vi "GUI_HTT_Switcher.vi"() -> ()   [LabVIEW 2013]
uses:
  Shared/GUI_Template/GUI_master/tcp_new_data_event.ctl
  Shared/GUI_Template/GUI_master/tcp new data cluster.ctl
panel:
  in  "DigitalOutput.Channel 2::1":enum16{"on", "off"}(ring) caption="Phosphor"
  in  "Phosphor":bool
  in  "DigitalOutput.Channel 1::1":enum16{"on", "off"}(ring)
  in  "DigitalOutput.Channel 0::1":enum16{"on", "off"}(ring) caption="Flipper"
  in  "Flipper":bool
  out "error IO 2":errorcluster
  out "fire::10":string
  out "tcp data event":T1
  in  "UDP error message":string
  in  "GUIdevice 2":string
  in  "GUIdevice 1":string="HTT-Switch-DAQPad"
  in  "stop":bool
  # "Energy"
  # "HTT Switcher"
  # "In"
  # "Out"
  # "In"
  # "Out"
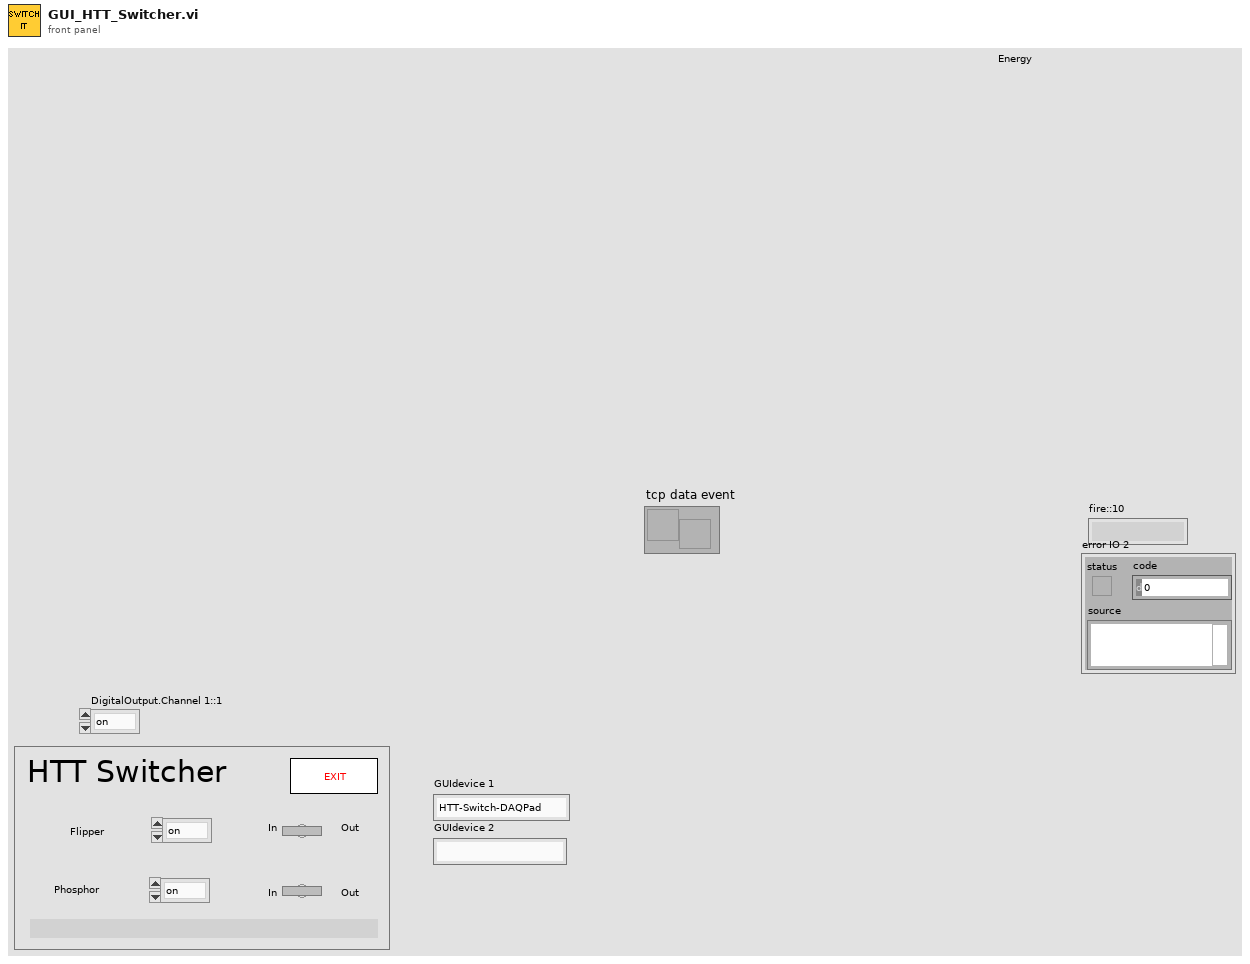
[diagram p1: front panel]
types:
  T1 = typedef "tcp_new_data_event.ctl" = refnum<user-event>
  T2 = typedef "tcp new data cluster.ctl" = cluster{"EventEnum":enum16{"new data", "connection status update"}, "Device name":string}
  T3 = enum32{"invalid app kind", "Development System", "Run Time System", "Student Edition", "Embedded LabVIEW", "Evaluation", "Custom"}
  T4 = enum32{"Invalid", "Standard", "Closed", "Hidden", "Minimized", "Maximized"}
  T5 = cluster{"Core":cluster{"Current VI Reference":refnum<vi>, "Close Panel on Exit?":bool}, "Heater timing offset":dbl, "Discharge timing offset":dbl, "Flipper":bool, "Tik1":u32, "Tik2":u32, "Flipperi":bool, "Phosphor":bool, "DigitalOutput.Channel 2::1":enum16{"on", "off"}}
  T6 = cluster{"Current VI Reference":refnum<vi>, "Close Panel on Exit?":bool}
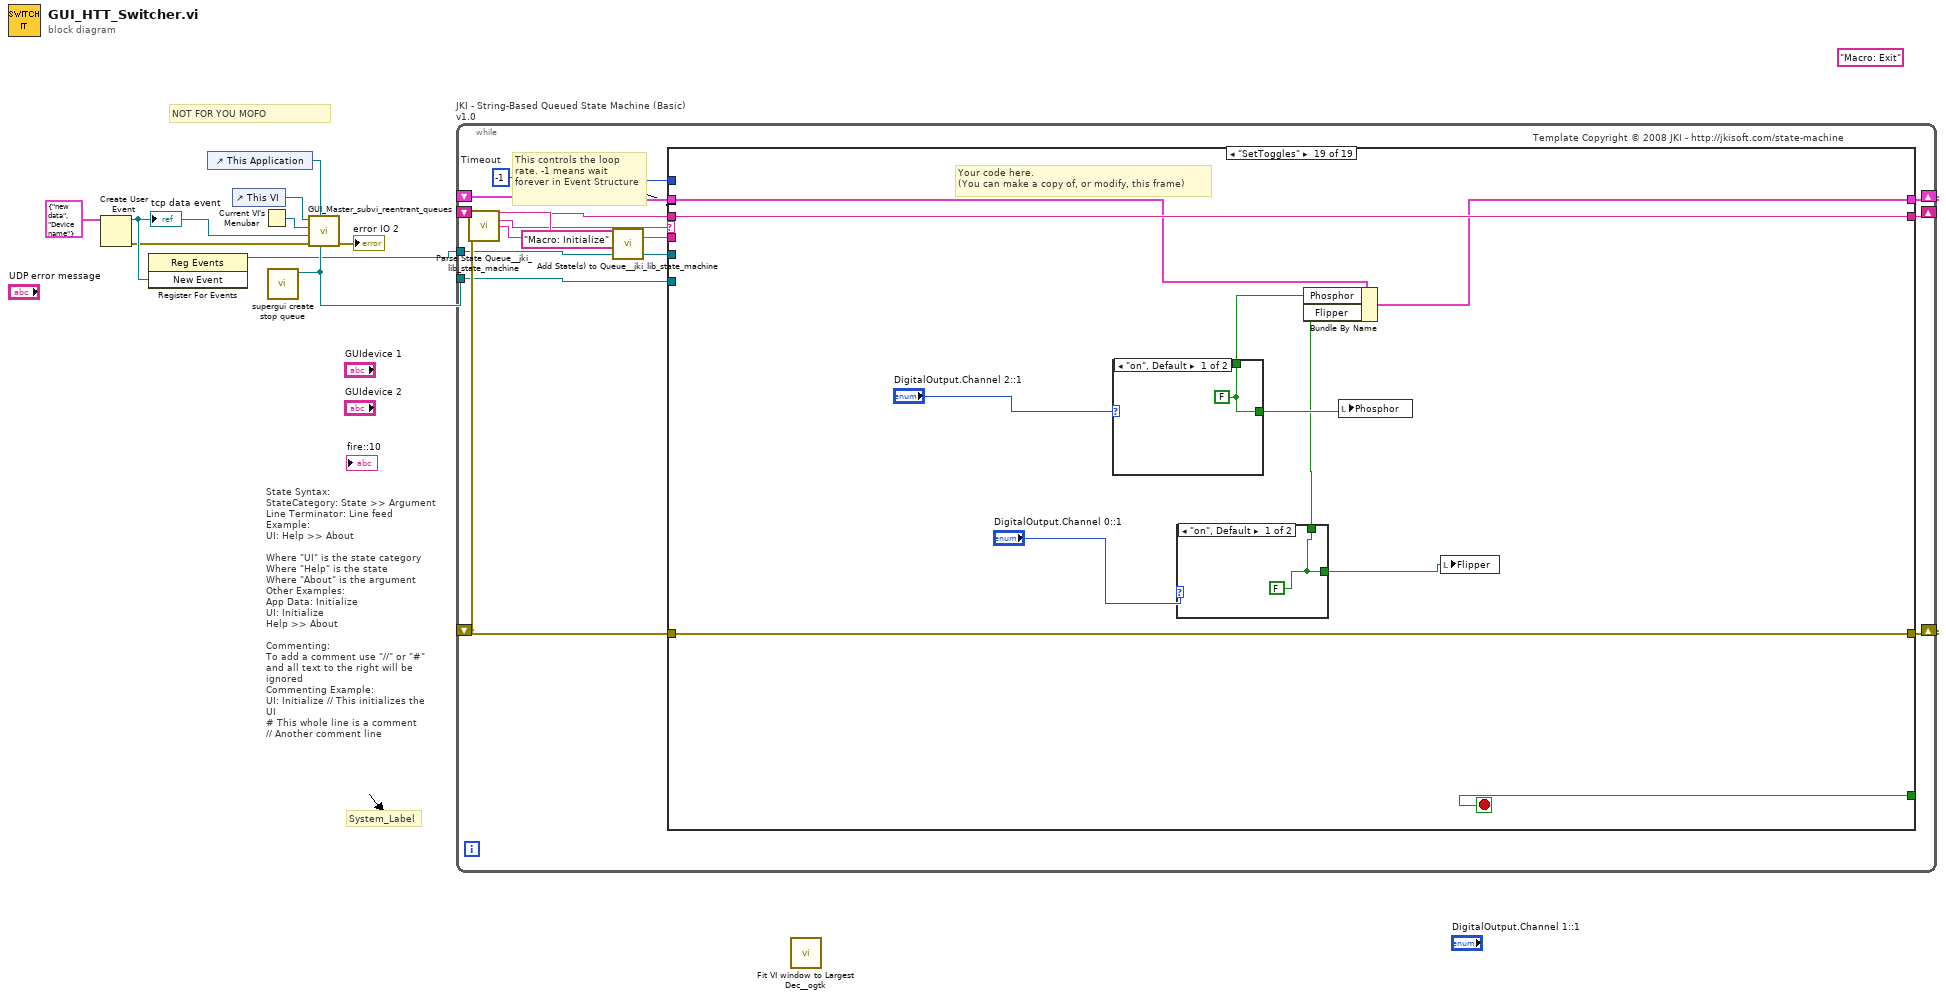
[diagram p0: block diagram]
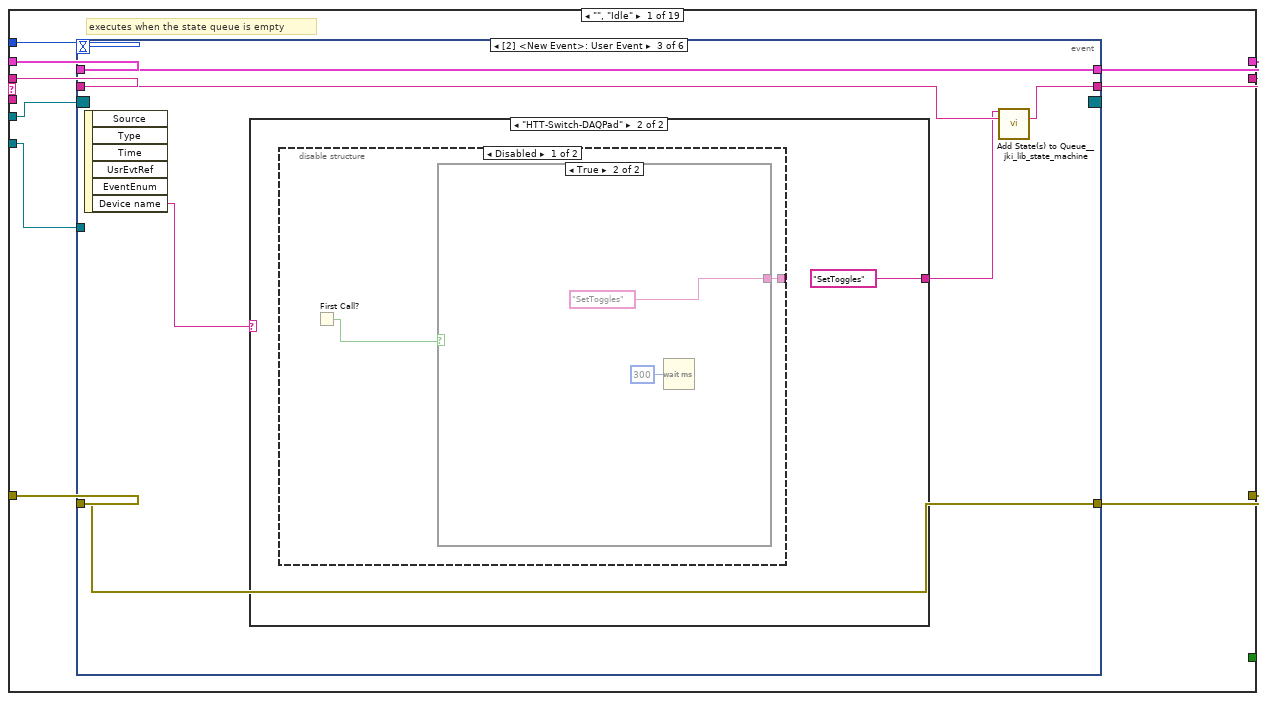
[diagram p2: hidden frame]
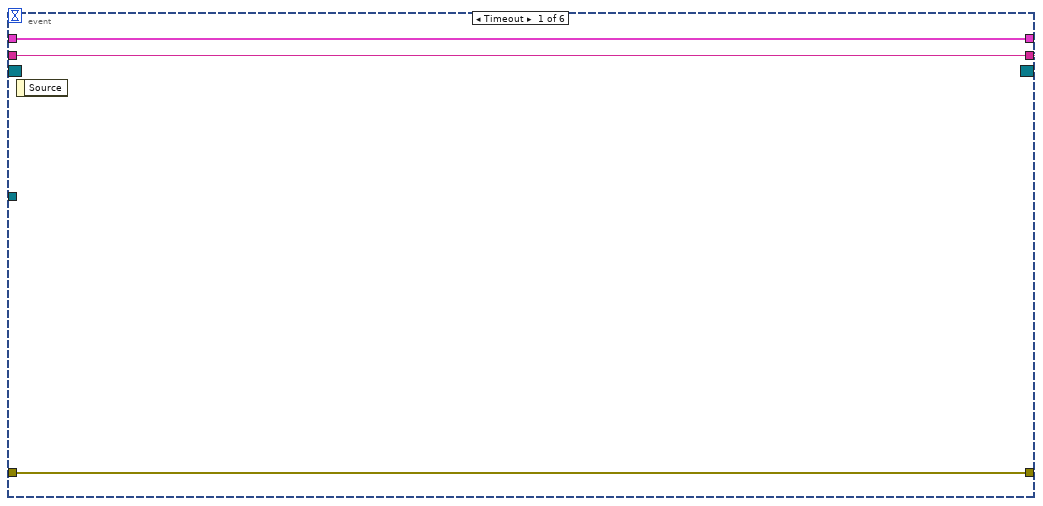
[diagram p3: hidden frame]
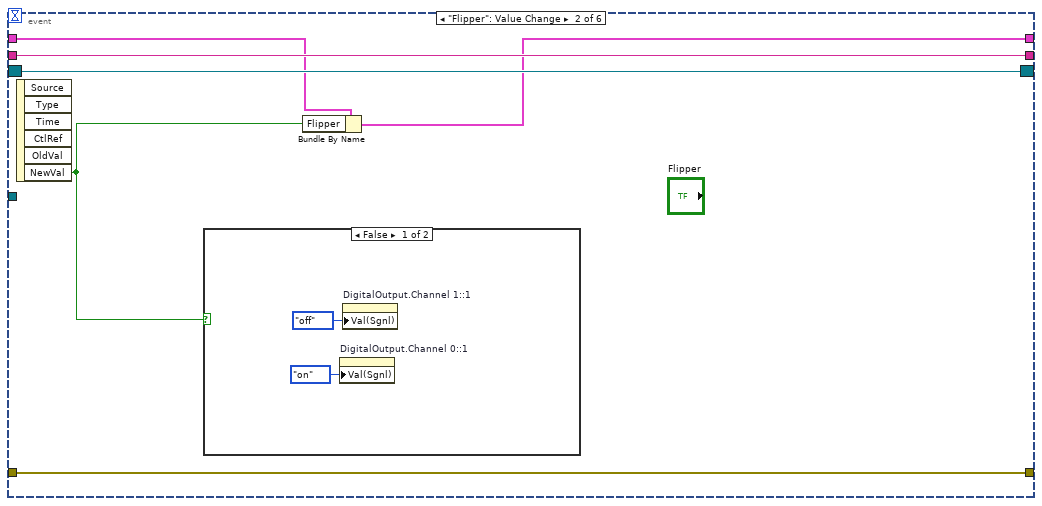
[diagram p4: hidden frame]
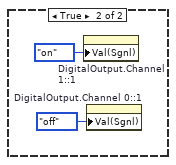
[diagram p5: hidden frame]
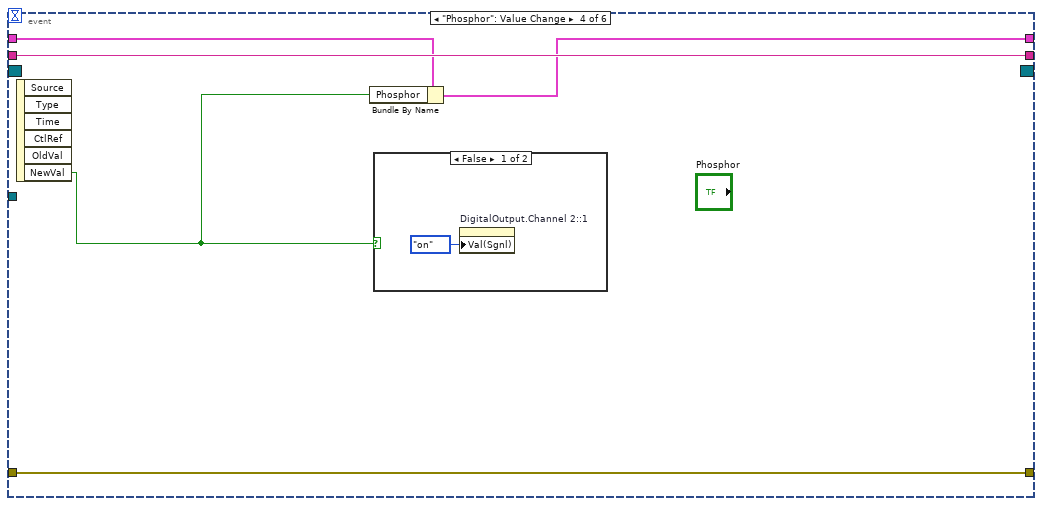
[diagram p9: hidden frame]
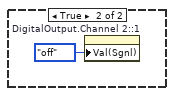
[diagram p10: hidden frame]
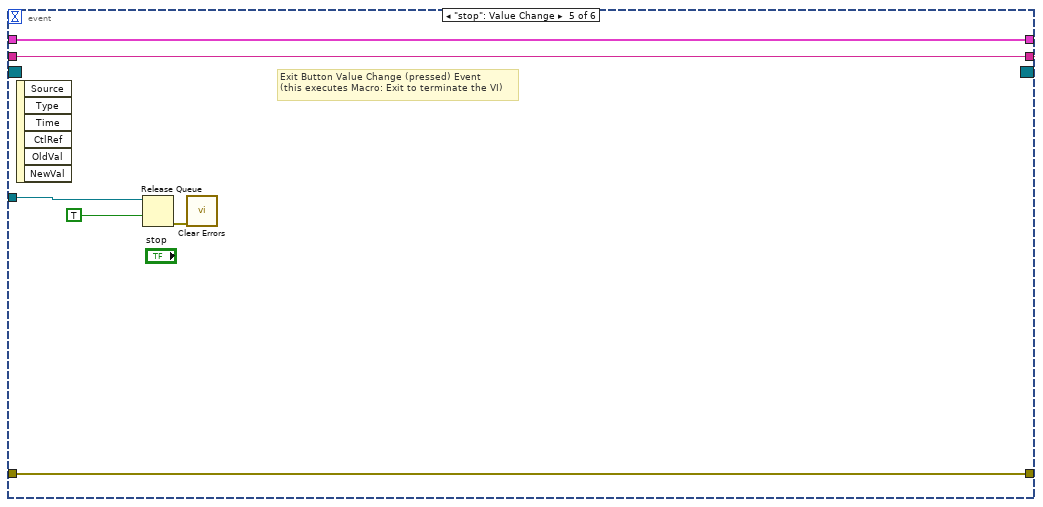
[diagram p11: hidden frame]
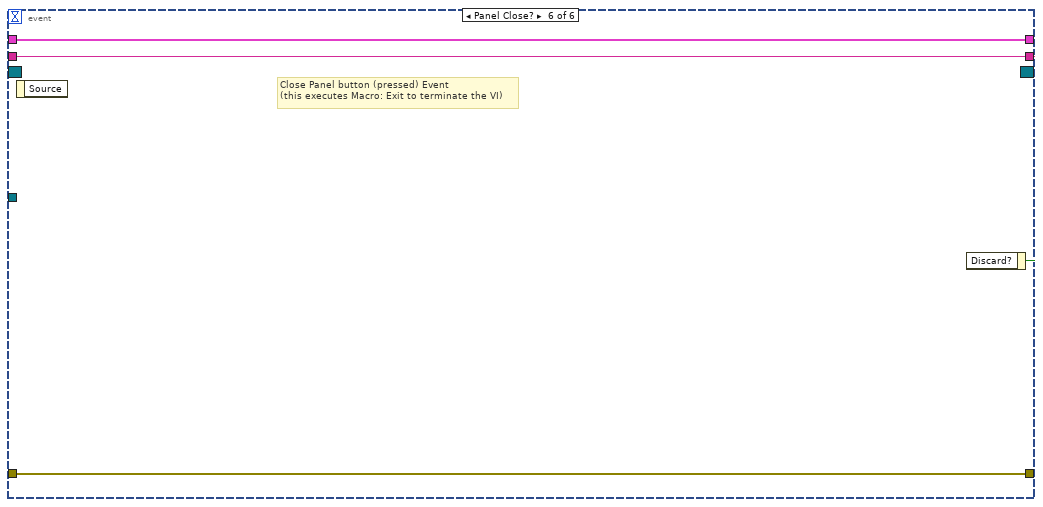
[diagram p12: hidden frame]
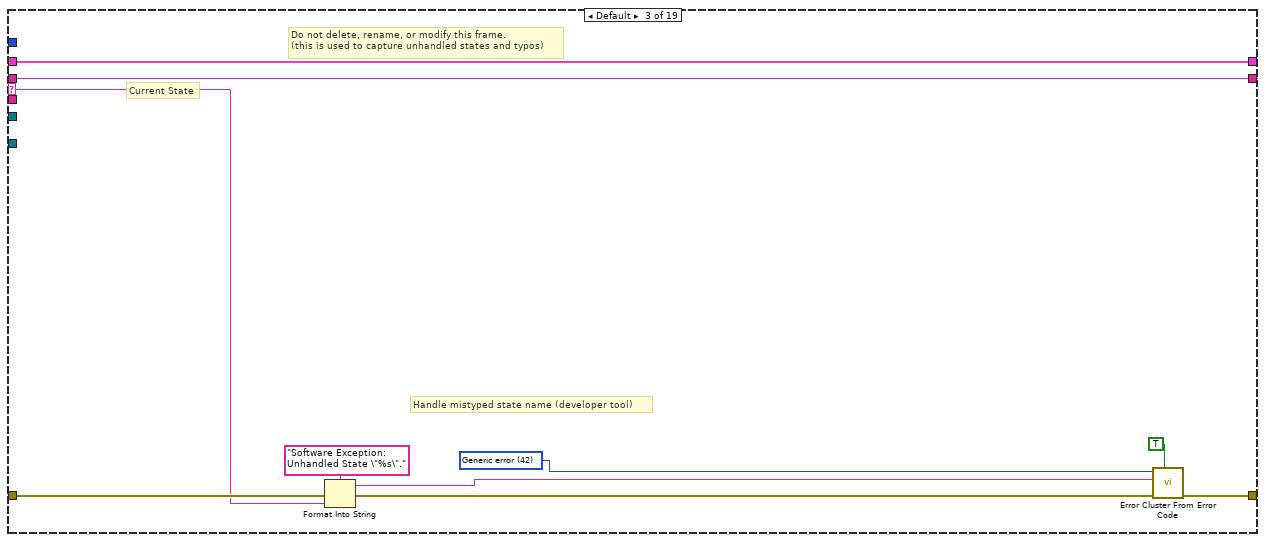
[diagram p14: hidden frame]
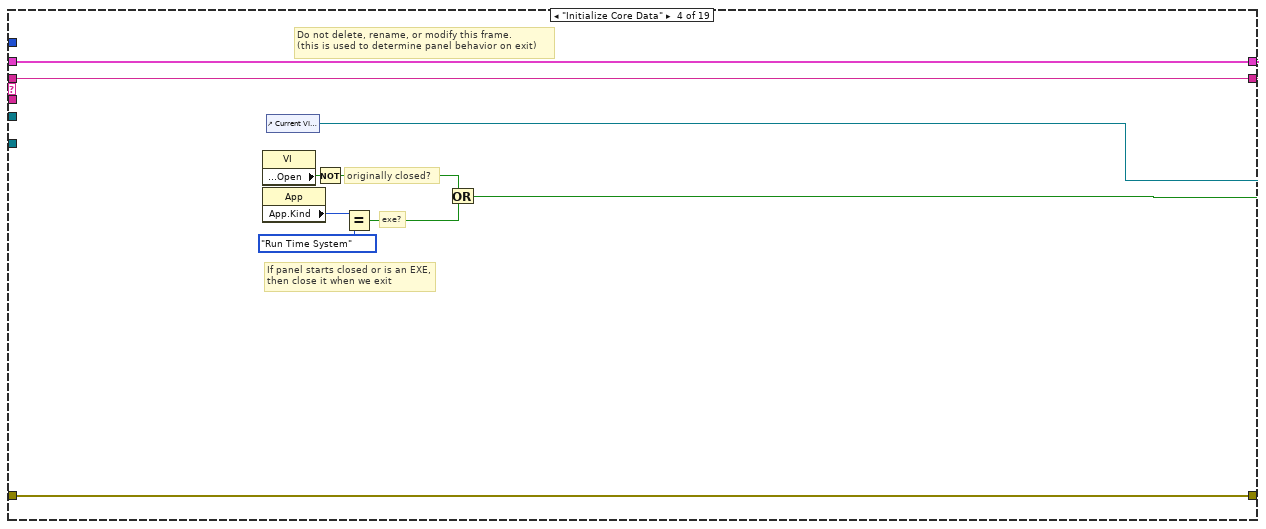
[diagram p15: hidden frame]
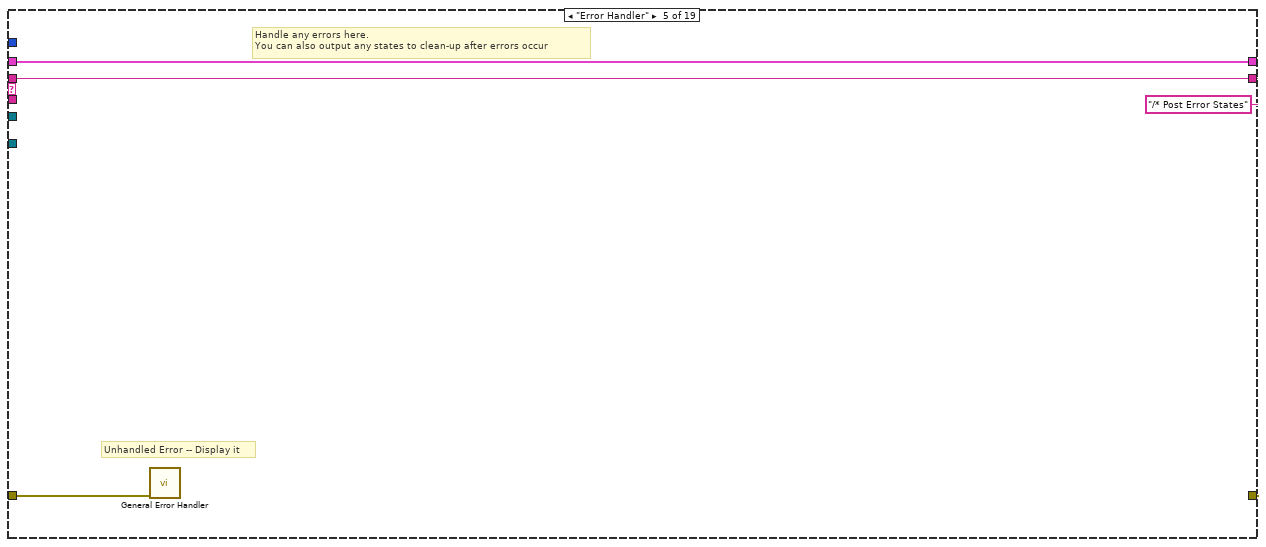
[diagram p16: hidden frame]
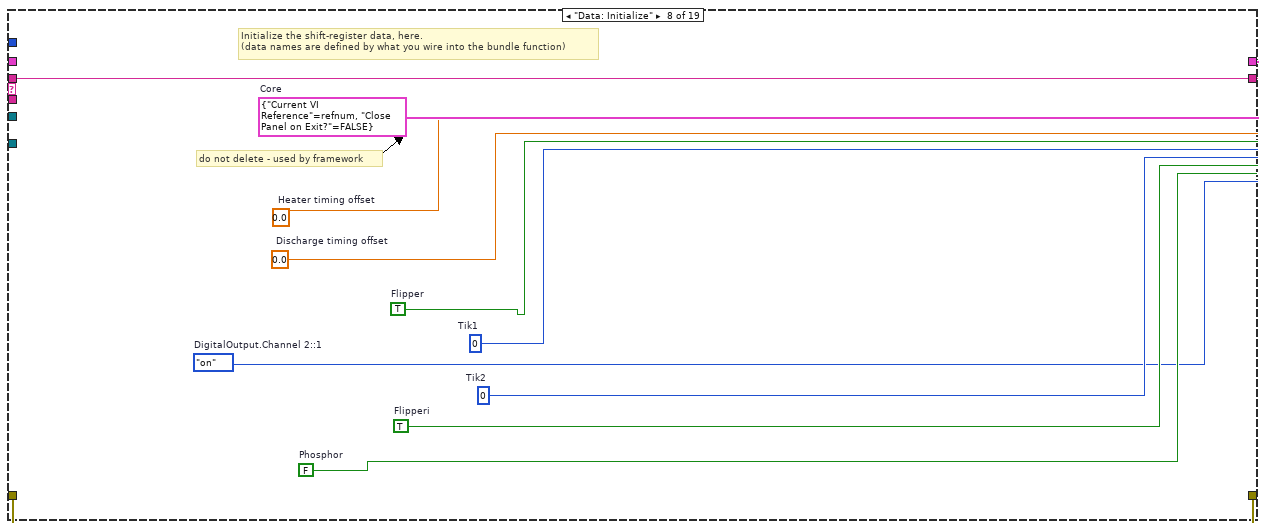
[diagram p19: hidden frame]
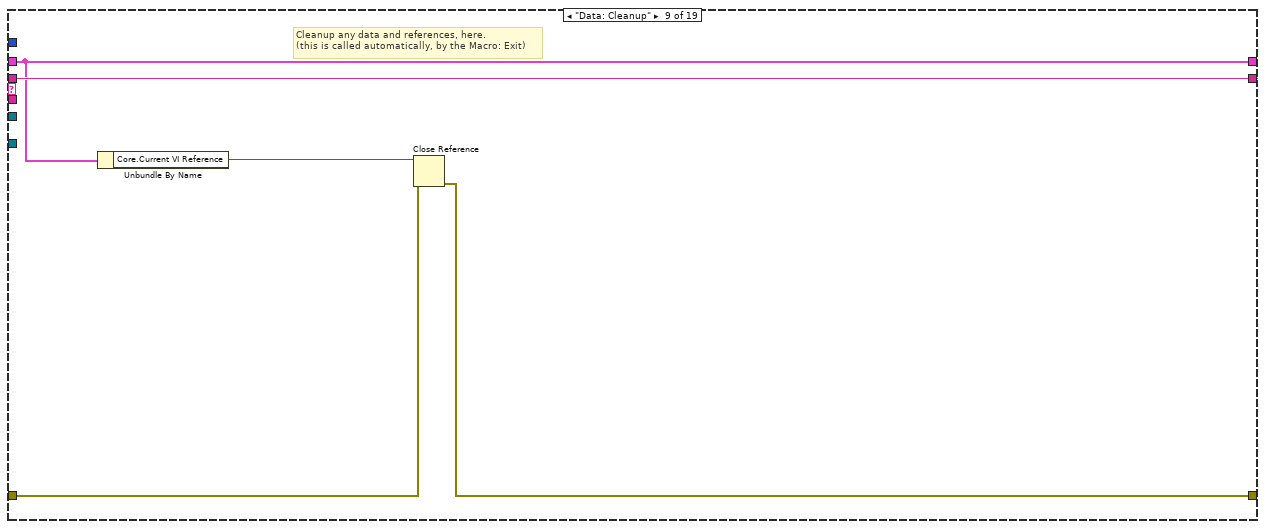
[diagram p20: hidden frame]
diagram:
  (unwired) "Macro: Exit"
  # "State Syntax:\nStateCategory: State >> Argument\nLine Terminator: Line feed\nExample:\nUI: Help >> About\n\nWhere \"UI\" is the state category\nWhere \"Help\" is the state\nWhere \"About\" is the argument\nOther Examples:\nApp Data: Initialize\nUI: Initialize\nHelp >> About\n\nCommenting:\nTo add a comment use \"//\" or \"#\" and all text to the right will be ignored\nCommenting Example:\nUI: Initialize // This initializes the UI\n# This whole line is a comment\n// Another comment line"
  # "This controls the loop rate. -1 means wait forever in Event Structure"
  # "System_Label"
  # "NOT FOR YOU MOFO"
  n1 = Create User Event(user event datatype=T2 {"EventEnum"=enum."new data", "Device name"="Device name"} ("New Event")) -> (user event=w10:refnum<user-event>, error out=w9:errorcluster)  [unwired: 1 in]
  "tcp data event" <- w10
  n2 = register-events(w10) -> (reference out=w1:refnum<event-registration>)  [unwired: 2 in, 1 out]
  n3 = control-ref of="This Application"() -> (w11:refnum<vi>)
  n4 = control-ref of="This VI"() -> (w5:refnum<vi>)
  n5 = Current VI's Menubar() -> (w7:refnum<k9>)
  n6 = call "supergui create stop queue.vi"() -> ("STOP Queue out"=w2:refnum<queue>)  [unwired: 11 in]
  n7 = call "GUI_Master_subvi_reentrant_queues.vi"("STOP Queue in"=w2, "This Application"=w11, "error in (no error)"=w9, "tcp data event"=w10, "Caller menu reference"=w7, "Caller VI ref"=w5) -> ("error out"=→"error IO 2":errorcluster)  [unwired: 5 in]
  n8 = call <vilib>:"Add State(s) to Queue__jki_lib_state_machine.vi"("State(s) in (\"\")"="Macro: Initialize") -> ("States Out"=w3:string)  [unwired: 14 in]
  n9 = while "JKI - String-Based Queued State Machine (Basic) v1.0" {
    shift-right: [w17] -> _
    shift-left: _ -> [w16]
    shift-right: [w20] -> _
    shift-left: _ -> [w14]
    shift-right: [w19] -> _
    shift-left: w3 -> [w21]
    tunnel: w1 -> [w13]
    tunnel: w2 -> [w12]
    stop <- w18 stop-if-true
    w15 = -1  # Timeout
    # "Template Copyright © 2008 JKI - http://jkisoft.com/state-machine"
    n10 = call <vilib>:"Parse State Queue__jki_lib_state_machine.vi"("State Queue"=w21, "Error In (no error)"=w14) -> ("Remaining States"=w23:string, "Current State"=w24:string, "Arguments"=w22:string)  [unwired: 11 in]
    n11 = case shown="\"SetToggles\"" w24 {
      selector: w24 -> [_ _ w84 _ _ _ _ _ _ _ _ _ _ _ _ _ _ _ _]
      tunnel: w23 -> [w33 w83 w88 w106 w112 w117 w121 w134 w140 w144 w148 w154 w165 w191 w196 w206 w210 w216 w227]
      tunnel: w22 -> [_ _ _ _ _ _ _ _ _ _ _ w149 w159 _ _ _ _ _ _]
      tunnel: w16 -> [w31 w80 w86 w97 w109 w115 w118 _ w135 w141 w146 w152 w161 w188 w192 w203 w207 w214 w220]
      tunnel: [w30 w81 w90 w103 errorcluster {"status"=FALSE, "code"=0, "source"=""} ("error out") w114 w119 w131 w136 w142 w145 w150 w162 w189 w194 w204 w208 w211 w223] -> w20
      tunnel: w14 -> [w29 w81 w89 w103 w108 w114 w119 w131 w137 w142 w145 w151 w163 w189 w194 w204 w208 w212 w223]
      tunnel: [w32 w82 w87 w105 w111 w116 w120 w133 w139 w143 w147 w153 w164 w190 w195 w205 w209 w215 w226] -> w19
      tunnel: [_ _ _ _ _ TRUE _ _ _ _ _ _ _ _ _ _ _ _ _] -> w18
      tunnel: [w25 w80 w86 w104 w109 w115 w118 w132 w135 w141 w146 w152 w161 w188 w192 w203 w207 w214 w219] -> w17
      tunnel: w15 -> [w28 _ _ _ _ _ _ _ _ _ _ _ _ _ _ _ _ _ _]
      tunnel: w13 -> [w27 _ _ _ _ _ _ _ _ _ _ _ _ _ _ _ _ _ _]
      tunnel: w12 -> [w26 _ _ _ _ _ _ _ _ _ _ _ _ _ _ _ _ _ _]
      frame "", "Idle" {
        # "executes when the state queue is empty"
        n12 = event shown="[2] <New Event>: User Event" {
          selector: w27 -> [_ w42 _ _ _ _]
          dyn-events: [_ w42 _ _ _ _] -> _
          timeout: w28 -> [_ _ _ _ _ _]
          tunnel: w33 -> [w37 w43 w50 w63 w73 w79]
          tunnel: [w36 w43 w49 w63 w72 w78] -> w32
          tunnel: w31 -> [w34 w39 w52 w61 w70 w76]
          tunnel: [w35 w41 w51 w62 w71 w77] -> w30
          tunnel: w29 -> [w35 w41 w51 w62 w71 w77]
          tunnel: w26 -> [_ _ _ _ w67 _]
          tunnel: [w34 w38 w52 w60 w70 w76] -> w25
          event Timeout {
            n13 = event-data() -> ()  [unwired: 1 in, 1 out]
            n14 = call <vilib>:"Add State(s) to Queue__jki_lib_state_machine.vi"("State(s) in (\"\")"=w37) -> ("States Out"=w36:string)  [unwired: 14 in]
          }
          event "Flipper": Value Change {
            n15 = event-data() -> ("NewVal"=w40:bool)  [unwired: 1 in, 5 out]
            n16 = case shown="False" w40 {
              frame False {
                n17 = property on="DigitalOutput.Channel 0::1" class="Enum (strict)"("Val(Sgnl)"=enum16{"on", "off"}."on" ("Value (Signaling)")) -> ()  [unwired: 2 in, 2 out]
                n18 = property on="DigitalOutput.Channel 1::1" class="Enum (strict)"("Val(Sgnl)"=enum16{"on", "off"}."off" ("Value (Signaling)")) -> ()  [unwired: 2 in, 2 out]
              }
              frame True {
                n19 = property on="DigitalOutput.Channel 1::1" class="Enum (strict)"("Val(Sgnl)"=enum16{"on", "off"}."on" ("Value (Signaling)")) -> ()  [unwired: 2 in, 2 out]
                n20 = property on="DigitalOutput.Channel 0::1" class="Enum (strict)"("Val(Sgnl)"=enum16{"on", "off"}."off" ("Value (Signaling)")) -> ()  [unwired: 2 in, 2 out]
              }
            }
            n21 = Bundle By Name(cluster=w39, "Flipper"=w40) -> (w38:T5)
          }
          event User Event {
            n22 = event-data() -> ("Device name"=w53:string)  [unwired: 1 in, 5 out]
            n23 = case shown="\"HTT-Switch-DAQPad\"" w53 {
              tunnel: [_ "SetToggles"] -> w48
              frame "False", Default {
              }
              frame "HTT-Switch-DAQPad" {
                n24 = disable-structure shown="Disabled" {
                  disable-tunnel: [w55 _] -> _
                  frame Disabled {
                    n25 = First Call?() -> (First Call?: T/F=w56:bool)
                    n26 = case shown="True" w56 {
                      tunnel: [_ "SetToggles"] -> w55
                      frame False {
                      }
                      frame True {
                        n27 = Wait (ms)(milliseconds to wait=u32 300) -> ()  [unwired: 1 out]
                      }
                    }
                  }
                  frame Enabled {
                  }
                }
              }
            }
            n28 = call <vilib>:"Add State(s) to Queue__jki_lib_state_machine.vi"("State(s) in Front (\"\")"=w48, "State(s) in (\"\")"=w50) -> ("States Out"=w49:string)  [unwired: 13 in]
          }
          event "Phosphor": Value Change {
            n29 = event-data() -> ("NewVal"=w59:bool)  [unwired: 1 in, 5 out]
            n30 = Bundle By Name(cluster=w61, "Phosphor"=w59) -> (w60:T5)
            n31 = case shown="False" w59 {
              frame False {
                n32 = property on="DigitalOutput.Channel 2::1" class="Enum (strict)"("Val(Sgnl)"=enum16{"on", "off"}."on" ("Value (Signaling)")) -> ()  [unwired: 2 in, 2 out]
              }
              frame True {
                n33 = property on="DigitalOutput.Channel 2::1" class="Enum (strict)"("Val(Sgnl)"=enum16{"on", "off"}."off" ("Value (Signaling)")) -> ()  [unwired: 2 in, 2 out]
              }
            }
          }
          event "stop": Value Change {
            # "Exit Button Value Change (pressed) Event\n(this executes Macro: Exit to terminate the VI)"
            n34 = event-data() -> ()  [unwired: 1 in, 6 out]
            n35 = Release Queue(queue=w67, force destroy? (F)=TRUE) -> (error out=w68:errorcluster)  [unwired: 1 in, 2 out]
            n36 = call <vilib>:"Clear Errors.vi"("error in (no error)"=w68) -> ()  [unwired: 6 in, 1 out]
            n37 = call <vilib>:"Add State(s) to Queue__jki_lib_state_machine.vi"("State(s) in Front (\"\")"="Macro: Exit", "State(s) in (\"\")"=w73) -> ("States Out"=w72:string)  [unwired: 13 in]
          }
          event Panel Close? {
            # "Discard the event because we'll close the front panel ourselves in Macro: Exit"
            # "Close Panel button (pressed) Event\n(this executes Macro: Exit to terminate the VI)"
            n38 = event-data() -> ()  [unwired: 1 in, 1 out]
            n39 = event-data("Discard?"=TRUE) -> ()  [unwired: 1 in, 1 out]
            n40 = call <vilib>:"Add State(s) to Queue__jki_lib_state_machine.vi"("State(s) in Front (\"\")"="Macro: Exit", "State(s) in (\"\")"=w79) -> ("States Out"=w78:string)  [unwired: 13 in]
          }
        }
      }
      frame "---------- Core ----------" {
        # "Do not put any code in this frame.\n(it is a separator no-op)"
        n41 = call <vilib>:"Add State(s) to Queue__jki_lib_state_machine.vi"("State(s) in (\"\")"=w83) -> ("States Out"=w82:string)  [unwired: 14 in]
      }
      frame Default {
        w93 = 42 items=["No error", "Argument error", "Memory is full", "Out of zone", "End of file", "File already open", "Generic file I/O error", "File not found", "File permission error", "Disk is full", "Duplicate path", "Too many files open", "System feature not enabled", "Resource file not found", "Cannot add resource", "Resource not found", "Image not found", "Image memory error", "Pen does not exist", "Config type invalid", "Config token not found", "Config parse error", "Config memory error", "Bad external code format", "Bad external code offset", "External code not present", "Null window", "Destroy window error", "Null menu", "Print aborted", "Bad print record", "Print driver error", "Windows error during printing", "Memory error during printing", "Print dialog error", "Generic print error", "Invalid device refnum", "Device not found", "Device parameter error", "Device unit error", "Cannot open device", "Device call aborted", "Generic error", "Cancelled by user", "Object ID too low", "Object ID too high", "Object not in heap", "Unknown heap", "Unknown object (invalid DefProc)", "Unknown object (DefProc not in table)", "Message out of range", "Invalid (null) method", "Unknown message", "Manager call not supported", "Bad address", "Network operation in progress", "Network operation timed out", "Connection is busy", "Network attribute not supported", "Network error", "Address in use", "System out of memory", "Connection aborted", "Connection refused", "Not connected", "Already connected", "Connection closed", "Initialization error (interapplication manager)", "Bad occurrence", "Wait on unbound occurrence handler", "Occurrence queue overflow", "Datalog type conflict", "Unused", "Unrecognized type (interapplication manager)", "Memory corrupt", "Failed to make temporary DLL", "Old CIN version", "Drag socket not found", "Failed to load drop-object", "Failed to register OLE object", "Failed to release OLE object", "Format specifier type mismatch", "Unknown format specifier", "Too few format specifiers", "Too many format specifiers", "Scan failed", "Newer CIN version", "Error converting to variant", "Runtime menu error", "Password tampered", "Variant attribute not found", "Incompatible variant data type", "Event data is not available", "Event Store is not present", "Occurrence is not found", "Event Queue is not created", "Event info is not available", "Refnum passed is NULL", "Error retrieving Class GUID", "Error retrieving CoClass GUID", "Error retrieving TypeLib GUID.", "Bad built application magic bytes.", "Specific driver is different from the specific driver associated with the Logical Name.", "There is no session opened to the class driver.", "Max Error", "MAX - Error with config objects", "MAX - Error loading configuration", "MAX - Group not supported"]
        # "Current State"
        # "Do not delete, rename, or modify this frame.\n(this is used to capture unhandled states and typos)"
        # "Handle mistyped state name (developer tool)"
        n42 = Format Into String(format string="Software Exception: Unhandled State \"%s\"." ("message"), error in=w89, w84) -> (resulting string=w92:string, error out=w91:errorcluster)  [unwired: 1 in]
        n43 = call <vilib>:"Error Cluster From Error Code.vi"("show call chain? (False)"=TRUE, "error in (no error)"=w91, "error message (\"\")"=w92, "error code (0)"=w93) -> ("error out"=w90:errorcluster)  [unwired: 5 in]
        n44 = call <vilib>:"Add State(s) to Queue__jki_lib_state_machine.vi"("State(s) in (\"\")"=w88) -> ("States Out"=w87:string)  [unwired: 14 in]
      }
      frame "Initialize Core Data" {
        # "Do not delete, rename, or modify this frame.\n(this is used to determine panel behavior on exit)"
        # "originally closed?"
        # "exe?"
        # "If panel starts closed or is an EXE, then close it when we exit"
        n45 = property class="VI"() -> ("Front Panel.Open"=w102:bool)  [unwired: 2 in, 2 out]
        n46 = property class="App"() -> ("App.Kind"=w101:T3)  [unwired: 2 in, 2 out]
        n47 = control-ref of="Current VI Reference"() -> (w95:refnum<vi>)
        n48 = Not(x=w102) -> (.not. x?=w99:bool)
        n49 = Equal?(x=w101, y=T3."Run Time System" ("Application:Kind")) -> (x = y?=w98:bool)
        n50 = Or(x=w99, y=w98) -> (x .or. y?=w96:bool)
        n51 = Bundle By Name(cluster=w97, "Core.Current VI Reference"=w95, "Core.Close Panel on Exit?"=w96) -> (w104:T5)
        n52 = call <vilib>:"Add State(s) to Queue__jki_lib_state_machine.vi"("State(s) in (\"\")"=w106) -> ("States Out"=w105:string)  [unwired: 14 in]
      }
      frame "Error Handler" {
        # "Unhandled Error -- Display it"
        # "Handle any errors here.\nYou can also output any states to clean-up after errors occur"
        # "Clear error"
        n53 = call <vilib>:"General Error Handler.vi"("error in (no error)"=w108) -> ()  [unwired: 10 in, 5 out]
        n54 = call <vilib>:"Add State(s) to Queue__jki_lib_state_machine.vi"("State(s) in Front (\"\")"="/* Post Error States", "State(s) in (\"\")"=w112) -> ("States Out"=w111:string)  [unwired: 13 in]
      }
      frame "Exit" {
        # "Do not put any code in this frame.\n(No errors that occur here will be handled.)"
        n55 = call <vilib>:"Add State(s) to Queue__jki_lib_state_machine.vi"("State(s) in (\"\")"=w117) -> ("States Out"=w116:string)  [unwired: 14 in]
      }
      frame "---------- Data ----------" {
        # "Do not put any code in this frame.\n(It is a separator no-op. You can make a copy of this frame to create a new Data frame)"
        n56 = call <vilib>:"Add State(s) to Queue__jki_lib_state_machine.vi"("State(s) in (\"\")"=w121) -> ("States Out"=w120:string)  [unwired: 14 in]
      }
      frame "Data: Initialize" {
        w122 = enum16{"on", "off"}."on"  # DigitalOutput.Channel 2::1
        w123 = FALSE  # Phosphor
        w124 = TRUE  # Flipper
        w125 = TRUE  # Flipperi
        w127 = u32 0  # Tik1
        w126 = u32 0  # Tik2
        w128 = 0.0  # Discharge timing offset
        w129 = 0.0  # Heater timing offset
        w130 = T6 {"Current VI Reference"=refnum, "Close Panel on Exit?"=FALSE}  # Core
        # "do not delete - used by framework"
        # "Expand Bundle to add new data elements to shift register data."
        # "Add new data here."
        # "Data names and types of shift register data are defined by this bundle."
        # "Initialize the shift-register data, here.\n(data names are defined by what you wire into the bundle function)"
        n57 = Bundle("Core"=w130, "Heater timing offset"=w129, "Discharge timing offset"=w128, "Flipper"=w124, "Tik1"=w127, "Tik2"=w126, "Flipperi"=w125, "Phosphor"=w123, "DigitalOutput.Channel 2::1"=w122) -> (w132:T5)  [unwired: 1 in]
        n58 = call <vilib>:"Add State(s) to Queue__jki_lib_state_machine.vi"("State(s) in (\"\")"=w134) -> ("States Out"=w133:string)  [unwired: 14 in]
      }
      frame "Data: Cleanup" {
        # "Cleanup any data and references, here.\n(this is called automatically, by the Macro: Exit)"
        n59 = Unbundle By Name(w135) -> ("Core.Current VI Reference"=w138:refnum<vi>)
        n60 = Close Reference(reference=w138, error in (no error)=w137) -> (error out=w136:errorcluster)
        n61 = call <vilib>:"Add State(s) to Queue__jki_lib_state_machine.vi"("State(s) in (\"\")"=w140) -> ("States Out"=w139:string)  [unwired: 14 in]
      }
      frame "---------- UI ----------" {
        # "Do not put any code in this frame.\n(It is a separator no-op. You can make a copy of this frame to create a new UI frame)"
        n62 = call <vilib>:"Add State(s) to Queue__jki_lib_state_machine.vi"("State(s) in (\"\")"=w144) -> ("States Out"=w143:string)  [unwired: 14 in]
      }
      frame "UI: Initialize" {
        # "Initialize the User Interface, here.\n(this is called automatically, by the Macro: Init)"
        n63 = call <vilib>:"Add State(s) to Queue__jki_lib_state_machine.vi"("State(s) in (\"\")"=w148) -> ("States Out"=w147:string)  [unwired: 14 in]
      }
      frame "UI: Cursor Set" {
        # "Argument"
        # "Set and Unset Cursor Busy.\n(Usage: \"UI: Cursor Set >> Busy|Idle\")"
        n64 = case shown="\"Idle\", Default" w149 {
          tunnel: w151 -> [w156 w158]
          tunnel: [w155 w157] -> w150
          frame "Idle", Default {
            n65 = call <vilib>:"Unset Busy.vi"("error in (no error)"=w156) -> ("error out"=w155:errorcluster)  [unwired: 10 in]
          }
          frame "Busy" {
            n66 = call <vilib>:"Set Busy.vi"("error in (no error)"=w158) -> ("error out"=w157:errorcluster)  [unwired: 9 in, 1 out]
          }
        }
        n67 = call <vilib>:"Add State(s) to Queue__jki_lib_state_machine.vi"("State(s) in (\"\")"=w154) -> ("States Out"=w153:string)  [unwired: 14 in]
      }
      frame "UI: Front Panel State" {
        # "Argument"
        # "Set Front Panel Open or Closed\n(Usage: \"UI: Front Panel State >> Open|Close\")"
        n68 = Unbundle By Name(w161) -> ("Core.Current VI Reference"=w160:refnum<vi>)
        n69 = case shown="\"Close\"" w159 {
          tunnel: w163 -> [w169 w182]
          tunnel: [w171 w183] -> w162
          tunnel: w160 -> [w170 w180]
          frame "Open", Default {
            n70 = property class="VI"(reference=w170, error in=w169) -> (reference out=w167:refnum<vi>, error out=w168:errorcluster, "Front Panel.Open"=w166:bool)
            n71 = case shown="False" w166 {
              tunnel: [w174 w177] -> w171
              tunnel: w168 -> [w173 w177]
              tunnel: w167 -> [w172 _]
              frame False {
                n72 = invoke class="VI" method="FP.Open"(reference=w172, error in=w173, "Activate"=TRUE, "State"=T4."Standard") -> (error out=w174:errorcluster)  [unwired: 1 in, 4 out]
              }
              frame True {
              }
            }
          }
          frame "Close" {
            n73 = property class="VI"(reference=w180, error in=w182) -> (reference out=w179:refnum<vi>, error out=w181:errorcluster, "Front Panel.Open"=w178:bool)
            n74 = case shown="True" w178 {
              tunnel: [w184 w187] -> w183
              tunnel: w181 -> [w184 w186]
              tunnel: w179 -> [_ w185]
              frame False {
              }
              frame True {
                n75 = invoke class="VI" method="FP.Close"(reference=w185, error in=w186) -> (error out=w187:errorcluster)  [unwired: 1 in, 2 out]
              }
            }
          }
        }
        n76 = call <vilib>:"Add State(s) to Queue__jki_lib_state_machine.vi"("State(s) in (\"\")"=w165) -> ("States Out"=w164:string)  [unwired: 14 in]
      }
      frame "---------- Macro ----------" {
        # "Do not put any code in this frame.\n(It is a separator no-op. You can make a copy of this frame to create a new Macro frame)"
        n77 = call <vilib>:"Add State(s) to Queue__jki_lib_state_machine.vi"("State(s) in (\"\")"=w191) -> ("States Out"=w190:string)  [unwired: 14 in]
      }
      frame "Macro: Initialize" {
        w193 = "Data: Initialize\nInitialize Core Data\nUI: Initialize\nUI: Front Panel State >> Open"  # Data: Initialize Initialize Core Data UI: Initialize UI: Front Panel State >> Open
        # "Initialization Macro\n(This is called once, when the VI starts)"
        n78 = call <vilib>:"Add State(s) to Queue__jki_lib_state_machine.vi"("State(s) in Front (\"\")"=w193, "State(s) in (\"\")"=w196) -> ("States Out"=w195:string)  [unwired: 13 in]
      }
      frame "Macro: Exit" {
        # "Exit Macro\n(This is called once, when the VI exits)"
        n79 = Unbundle By Name(w203) -> ("Core.Close Panel on Exit?"=w202:bool)
        n80 = Select(t="UI: Front Panel State >> Close", s=w202, f="") -> (s? t:f=w199:string)
        n81 = call <vilib>:"Add State(s) to Queue__jki_lib_state_machine.vi"("State(s) in (\"\")"=w199, "State(s) at Back (\"\")"="Data: Cleanup\nExit") -> ("States Out"=w197:string)  [unwired: 13 in]
        n82 = call <vilib>:"Add State(s) to Queue__jki_lib_state_machine.vi"("State(s) in Front (\"\")"=w197, "State(s) in (\"\")"=w206) -> ("States Out"=w205:string)  [unwired: 13 in]
      }
      frame "---------- New Category ----------" {
        # "Template Separator\n(You can make a copy of, or modify, this frame)"
        n83 = call <vilib>:"Add State(s) to Queue__jki_lib_state_machine.vi"("State(s) in (\"\")"=w210) -> ("States Out"=w209:string)  [unwired: 14 in]
      }
      frame "Action: Fire" {
        # "Your code here.\n(You can make a copy of, or modify, this frame)"
        n84 = property on="fire::10" class="Str"(error in=w212, "Val(Sgnl)"="fire>>force" ("Value (Signaling)")) -> (error out=w211:errorcluster)  [unwired: 1 in, 1 out]
        n85 = call <vilib>:"Add State(s) to Queue__jki_lib_state_machine.vi"("State(s) in (\"\")"=w216) -> ("States Out"=w215:string)  [unwired: 14 in]
      }
      frame "SetToggles" {
        # "Your code here.\n(You can make a copy of, or modify, this frame)"
        n86 = case shown="\"on\", Default" "DigitalOutput.Channel 2::1" {
          tunnel: [w230 w231] -> w224
          tunnel: [w230 w231] -> w218
          frame "on", Default {
            w230 = FALSE ("Phosphor")
          }
          frame "off" {
            w231 = TRUE ("Phosphor")
          }
        }
        n87 = case shown="\"on\", Default" "DigitalOutput.Channel 0::1" {
          tunnel: [w228 w229] -> w221
          tunnel: [w228 w229] -> w217
          frame "on", Default {
            w228 = FALSE ("Flipper")
          }
          frame "off" {
            w229 = TRUE ("Flipper")
          }
        }
        n88 = Bundle By Name(cluster=w220, "Phosphor"=w218, "Flipper"=w217) -> (w219:T5)
        n89 = local write "Phosphor"(w224) -> ()
        n90 = local write "Flipper"(w221) -> ()
        n91 = call <vilib>:"Add State(s) to Queue__jki_lib_state_machine.vi"("State(s) in (\"\")"=w227) -> ("States Out"=w226:string)  [unwired: 14 in]
      }
    }
  }
  n92 = call <userlib>:"Fit VI window to Largest Dec__ogtk.vi"() -> ()  [unwired: 6 in, 2 out]
